vi "BD_GUI_Actuatorcontrol_v1.vi"() -> ()   [LabVIEW 2016]
uses:
  Documents/Control 2.ctl
  <vilib>/Instr/_visa.llb/VISA Configure Serial Port (Instr).vi
panel:
  out "Output to Arduino:":string
  in  "?":bool
  in  "Desired Thickness:":ext caption="mm"
  out "Actuator 1:":T1 scale=15.0..950.0
  in  "stop":bool
  out "Analog value:":i32
  in  "flow control":u16(ring) items=["None"=0, "XON/XOFF"=1, "RTS/CTS"=2, "DTR/DSR"=4]
  in  "stop bits":u16(ring)=10 items=["1.0"=10, "1.5"=15, "2.0"=20]
  in  "parity":u16(ring) items=["None", "Odd", "Even", "Mark", "Space"]
  in  "data bits":u16=8 min=5 max=8 step=1
  in  "VISA resource name":refnum<visa-resource-name>="COM1"
  in  "baud rate":u32=9600
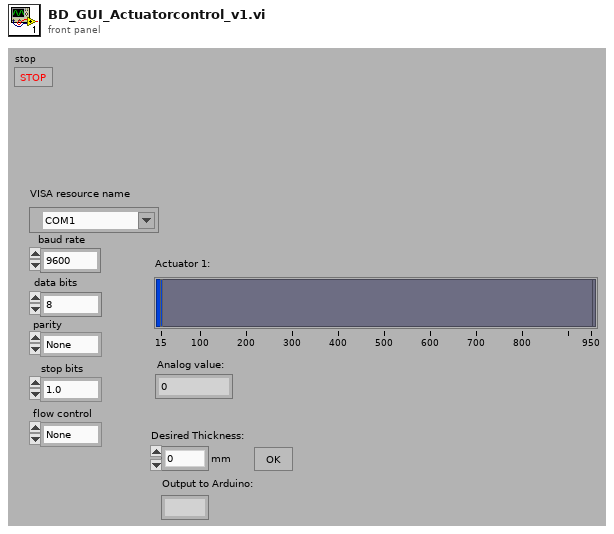
[diagram p1: front panel]
types:
  T1 = typedef "Control 2.ctl" = dbl
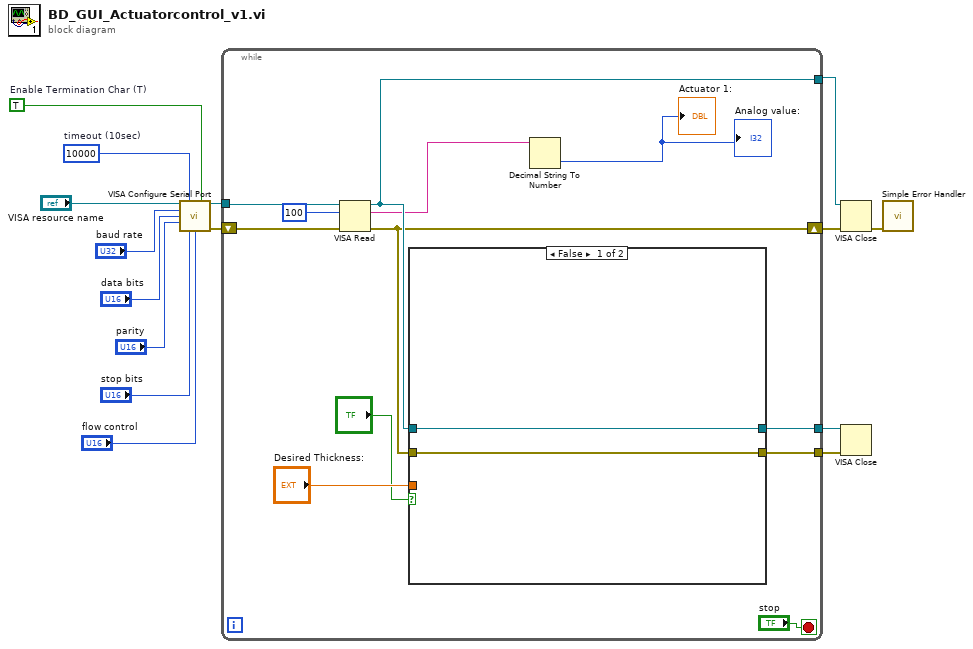
[diagram p0: block diagram]
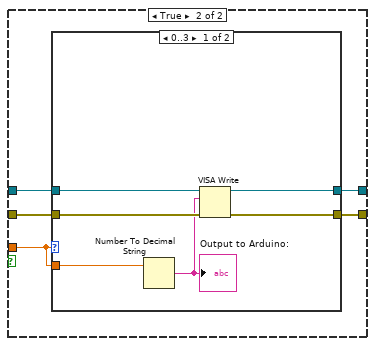
[diagram p2: hidden frame]
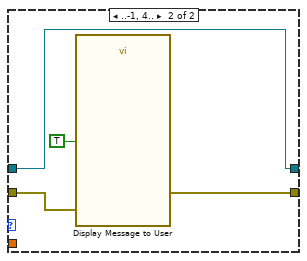
[diagram p3: hidden frame]
diagram:
  w8 = TRUE  # Enable Termination Char (T)
  w9 = u32 10000  # timeout (10sec)
  n1 = call-poly "VISA Configure Serial Port"("VISA resource name"="VISA resource name", "timeout (10sec)"=w9, "Enable Termination\nChar (T)"=w8, "baud rate (9600)"="baud rate", "data bits (8)"="data bits", "parity (0:none)"="parity", "stop bits (10: 1 bit)"="stop bits", "flow control (0:none)"="flow control") -> ("VISA resource name out"=w4:refnum<visa-resource-name>, "error out"=w15:errorcluster)  [unwired: 1 in, 5 out]
  n2 = while {
    tunnel: w4 -> [w21]
    shift-right: [w17] -> w14
    shift-left: w15 -> [w20]
    tunnel: [w26] -> w3
    tunnel: [w23] -> w2
    tunnel: [w22] -> w1
    stop <- "stop" stop-if-true
    n3 = VISA Read(VISA resource name=w21, byte count=100, error in (no error)=w20) -> (VISA resource name out=w26:refnum<visa-resource-name>, read buffer=w16:string, error out=w17:errorcluster)  [unwired: 1 out]
    n4 = case shown="False" "?" {
      tunnel: w17 -> [w29 w34]
      tunnel: w26 -> [w28 w33]
      tunnel: [w28 w32] -> w23
      tunnel: [w29 w31] -> w22
      tunnel: "Desired Thickness:" -> [_ w30]
      frame False {
      }
      frame True {
        n5 = case shown="0..3" w30 {
          tunnel: w34 -> [w40 w42]
          tunnel: w33 -> [w39 w43]
          tunnel: [w36 w43] -> w32
          tunnel: [w38 w44] -> w31
          tunnel: w30 -> [w37 _]
          frame 0..3 {
            n6 = Number To Decimal String(number=w37) -> (decimal integer string=w35:string)  [unwired: 1 in]
            "Output to Arduino:" <- w35
            n7 = VISA Write(VISA resource name=w39, write buffer=w35, error in (no error)=w40) -> (VISA resource name out=w36:refnum<visa-resource-name>, error out=w38:errorcluster)  [unwired: 1 out]
          }
          frame ..-1, 4.. {
            n8 = call "Display Message to User"("error in (no error)"=w42, "Enable"=TRUE) -> ("error out"=w44:errorcluster)  [unwired: 8 in, 1 out]
          }
        }
      }
    }
    n9 = Decimal String To Number(string=w16) -> (number=→"Analog value:" →"Actuator 1:":i32)  [unwired: 3 out]
  }
  n10 = VISA Close(VISA resource name=w3, error in (no error)=w14) -> (error out=w13:errorcluster)
  n11 = VISA Close(VISA resource name=w2, error in (no error)=w1) -> ()  [unwired: 1 out]
  n12 = call <vilib>:"Simple Error Handler.vi"("error in (no error)"=w13) -> ()  [unwired: 1 in, 8 out]
